vi "Czasomierz FVG.vi"(7 "Akcja (Wait)":T1=enum."Wait", 8 "error in (no error)":errorcluster, 10 "Czas (s)":dbl) -> (0 "error out":errorcluster, 2 "Elapsed?":bool, 3 "Elapsed Time":dbl)   [LabVIEW 2013]
uses:
  inne pliki/Akcje czas FVG.ctl
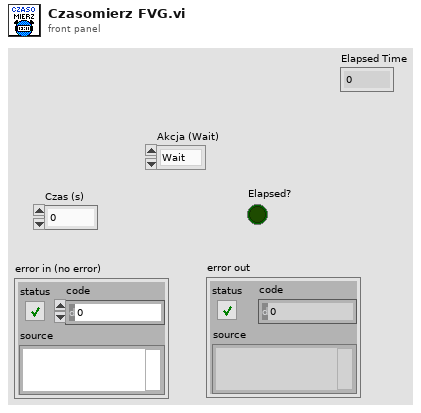
[diagram p1: front panel]
types:
  T1 = typedef "Akcje czas FVG.ctl" = enum16{"Reset", "Wait"}
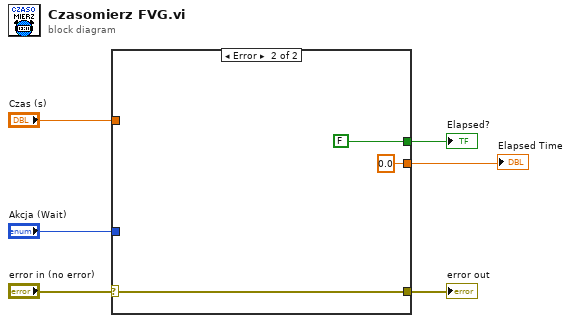
[diagram p0: block diagram]
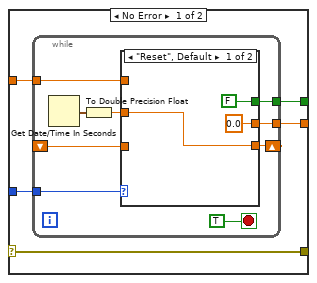
[diagram p2: hidden frame]
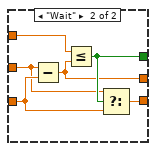
[diagram p3: hidden frame]
diagram:
  n1 = case shown="Error" "error in (no error)" {
    selector: "error in (no error)" -> [w8 w32]
    tunnel: "Akcja (Wait)" -> [w11 _]
    tunnel: "Czas (s)" -> [w10 _]
    tunnel: [w9 FALSE] -> w4
    tunnel: [w8 w32] -> w2
    tunnel: [w7 0.0] -> w1
    frame No Error {
      n2 = while {
        tunnel: w11 -> [w20]
        shift-right: [w16] -> _
        shift-left: _ -> [w15]
        tunnel: w10 -> [w14]
        tunnel: [w13] -> w9
        tunnel: [w12] -> w7
        stop <- TRUE stop-if-true
        n3 = Get Date/Time In Seconds() -> (seconds since 1Jan1904=w18:timestamp)
        n4 = To Double Precision Float(number=w18) -> (double precision float=w17:dbl)
        n5 = case shown="\"Reset\", Default" w20 {
          tunnel: w17 -> [w22 w25]
          tunnel: [w22 w26] -> w16
          tunnel: w15 -> [_ w27]
          tunnel: w14 -> [_ w29]
          tunnel: [FALSE w28] -> w13
          tunnel: [0.0 w24] -> w12
          frame "Reset", Default {
          }
          frame "Wait" {
            n6 = Subtract(x=w25, y=w27) -> (x-y=w24:dbl)
            n7 = Less Or Equal?(x=w29, y=w24) -> (x <= y?=w28:bool)
            n8 = Select(t=w25, s=w28, f=w27) -> (s? t:f=w26:dbl)
          }
        }
      }
    }
    frame Error {
    }
  }
  "Elapsed?" <- w4
  "error out" <- w2
  "Elapsed Time" <- w1
